vi "Construct_multipart_message_variant.vi"(0 "command":T3=enum."configure_rf", 1 "Command_Type":T1=enum."environment_control", 5 "parameters (JSON)":string="{\"invalid\":1}", 7 "datatype":T2, 9 "data in":variant, 11 "error in (no error)":errorcluster) -> (4 "Multipart message":string[](array[string]), 14 "Debug info":string, 15 "error out":errorcluster)   [LabVIEW 2019, in "mmW_commands.lvlib"]
uses:
  mmW_commands.lvlib
  TypeDefs/commands.ctl
  commands/typedefs/datatypes_.ctl
  TypeDefs/command_types.ctl
panel:
  out "type (none)":string="none"
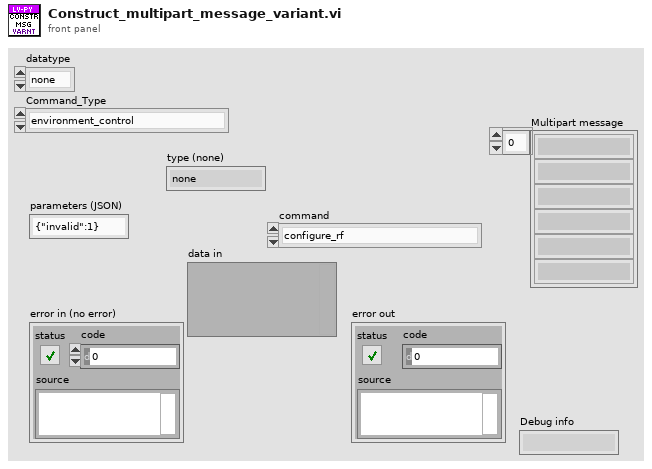
[diagram p1: front panel]
types:
  T1 = typedef "mmW_commands.lvlib/command_types.ctl" = enum16{"invalid_command", "instrument_control", "environment_control", "response"}
  T2 = typedef "mmW_commands.lvlib/datatypes_.ctl" = enum16{"none", "string", "interleaved_I16", "interleaved_I32", "I16_array", "I32_array", "JSONstring"}
  T3 = typedef "mmW_commands.lvlib/commands.ctl" = enum16{"configure_fs", "configure_rf", "configure_trigger", "equalization_enable", "equalization_start", "lo_sync_enable", "equalization_stop", "get_instrument_status", "get_versions", "initialize_hw", "pop_rx", "set_log_level", "Shutdown", "start", "start_instrument_app", "stop", "trans", "transceive", "trigger_burst", "trigger_sync_enable", "Write TX", "resp_generic", "resp_waveform", "send_trigger", "fetch", "transceive2"}
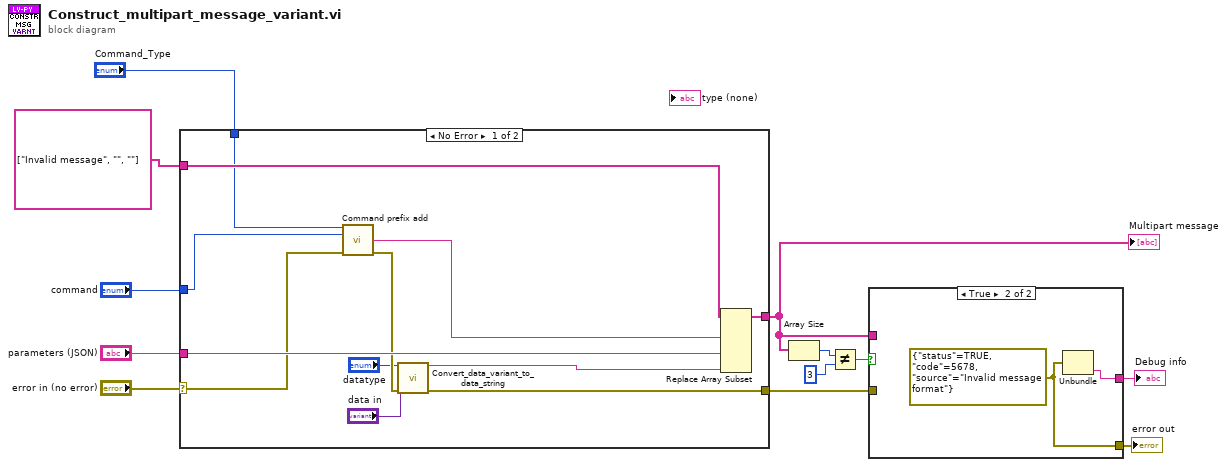
[diagram p0: block diagram]
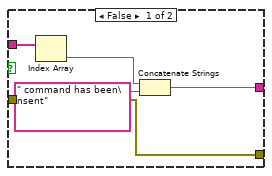
[diagram p2: hidden frame]
diagram:
  n1 = case shown="No Error" "error in (no error)" {
    selector: "error in (no error)" -> [w14 w25]
    tunnel: "parameters (JSON)" -> [w21 _]
    tunnel: [w19 w25] -> w5
    tunnel: [w24 w26] -> w4
    tunnel: string[] ["Invalid message", "", ""] -> [w23 w26]
    tunnel: "command" -> [w22 _]
    tunnel: "Command_Type" -> [w15 _]
    frame No Error {
      n2 = call "Command prefix add.vi"("Command_Types"=w15, "command"=w22, "error in (no error)"=w14) -> ("prefix+cmd"=w13:string, "error out"=w20:errorcluster)  [unwired: 10 in, 1 out]
      n3 = call "Convert_data_variant_to_data_string.vi"("datatype"="datatype", "data in"="data in", "error in (no error)"=w20) -> ("String"=w18:string, "error out"=w19:errorcluster)  [unwired: 11 in]
      n4 = Replace Array Subset(array=w23, new element #1=w13, new element #2=w21, new element #3=w18) -> (w24:string[])  [unwired: 3 in]
    }
    frame Error {
    }
  }
  "Multipart message" <- w4
  n5 = Array Size(array=w4) -> (size(s)=w9:i32)
  n6 = Not Equal?(x=w9, y=3) -> (x != y?=w7:bool)
  n7 = case shown="True" w7 {
    tunnel: [w31 w33] -> w6
    tunnel: w5 -> [w31 _]
    tunnel: w4 -> [w30 _]
    tunnel: [w27 w32] -> w3
    frame False {
      n8 = Index Array(array=w30) -> (element=w29:string)  [unwired: 1 in]
      n9 = Concatenate Strings(w29, " command has been\nsent" ("string")) -> (w27:string)
    }
    frame True {
      w33 = errorcluster {"status"=TRUE, "code"=5678, "source"="Invalid message format"} ("s? t:f")
      n10 = Unbundle(w33) -> ("source"=w32:string)  [unwired: 2 out]
    }
  }
  "error out" <- w6
  "Debug info" <- w3
